vi "save operation binary.vi"(8 "error in":errorcluster, 11 "state cluster":T1) -> (0 "error out":errorcluster, 3 "state out":T1)   [LabVIEW 2013, in "configuration library.lvlib"]
uses:
  configuration library.lvlib
  Controls/StateCluster.ctl
  <vilib>/NI/Tag Bus Data Framework/Configuration Editor/Classes/SystemConfigRepo/SystemConfigRepo.lvclass
  <vilib>/NI/Configuration Framework/Node/NodeRef.ctl
  <vilib>/NI/Configuration Framework/Node/NISE_CEF_Node.lvclass
  <vilib>/NI/Configuration Framework/Node/UserEventRef.ctl
  <vilib>/NI/Configuration Framework/Controls/EventCluster.ctl
  SplashScreen/splash screen.ctl
  SplashScreen/notifier data.ctl
  <vilib>/NI/Configuration Framework/hierarchy repo/NISE_CEF_HierarchyRepo.lvclass
  <vilib>/NI/Configuration Framework/tree serializer/NISE_CEF_TreeSerializer.lvlib
  <vilib>/NI/Configuration Framework/NISE_CEF_TreeControl.lvlib
  SplashScreen/splash screen.lvlib
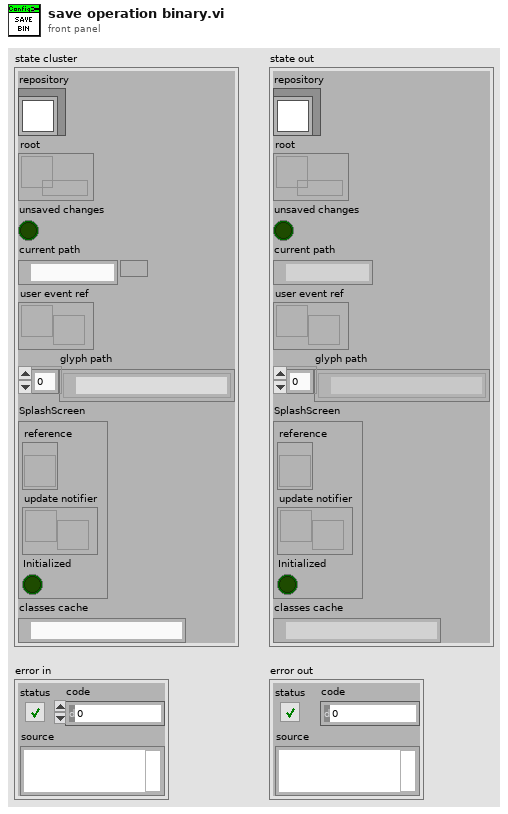
[diagram p1: front panel]
types:
  T1 = typedef "configuration library.lvlib/StateCluster.ctl" = cluster{"repository":refnum<class "SystemConfigRepo.lvclass">, "root":T2, "unsaved changes":bool, "current path":path, "user event ref":T3, "glyph path":path[], "SplashScreen":T4, "classes cache":path}
  T2 = typedef "NISE_CEF_Node.lvclass/NodeRef.ctl" = refnum<data-value>
  T3 = typedef "NISE_CEF_Node.lvclass/UserEventRef.ctl" = refnum<user-event>
  T4 = typedef "configuration library.lvlib/splash screen.lvlib/splash screen.ctl" = cluster{"reference":refnum<vi>, "update notifier":refnum<notifier>, "Initialized":bool}
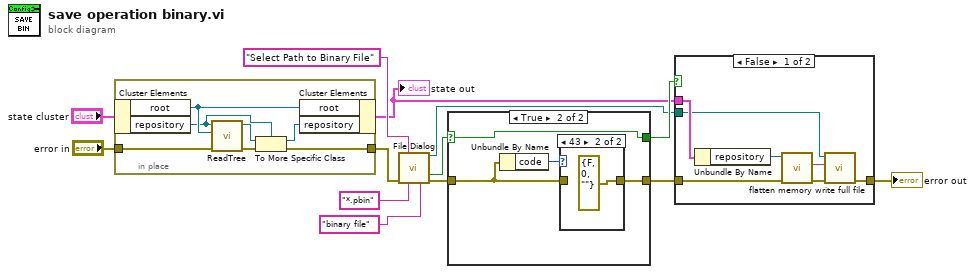
[diagram p0: block diagram]
diagram:
  n1 = in-place {
    in-place-border: "error in" -> [w20]
    in-place-border: [w17] -> w13
    n2 = in-place-cluster #1("state cluster") -> ("root"=w19:T2, "repository"=w15:refnum<class "SystemConfigRepo.lvclass">)
    n3 = call-dynamic "ReadTree.vi"("error in"=w20, "root"=w19, "repository in"=w15) -> ("error out"=w18:errorcluster, "repository out"=w16:refnum<class "NISE_CEF_Repository.lvclass">)  [unwired: 7 in]
    n4 = To More Specific Class(target class=w15, reference=w16, error in=w18) -> (specific class reference=w14:refnum<class "SystemConfigRepo.lvclass">, error out=w17:errorcluster)
    n5 = in-place-cluster #1("root"=w19, "repository"=w14) -> (w1:T1)
  }
  "state out" <- w1
  n6 = call "File Dialog"("prompt"="Select Path to Binary File" ("Prompt"), "error in"=w13, "pattern (all files)"="*.pbin" ("pattern"), "pattern label"="binary file") -> ("selected path"=w8:path, "cancelled"=w3:bool, "error out"=w2:errorcluster)  [unwired: 8 in, 1 out]
  n7 = case shown="True" w3 {
    selector: w3 -> [w21 w23]
    tunnel: w2 -> [w22 w25]
    tunnel: [w22 w24] -> w7
    tunnel: [w21 w23] -> w9
    frame False {
    }
    frame True {
      n8 = Unbundle By Name(w25) -> ("code"=w26:i32)
      n9 = case shown="43" w26 {
        tunnel: w25 -> [w27 _]
        tunnel: [w27 errorcluster {"status"=FALSE, "code"=0, "source"=""} ("error out")] -> w24
        frame Default {
        }
        frame 43 {
        }
      }
    }
  }
  n10 = case shown="False" w9 {
    tunnel: w1 -> [w35 _]
    tunnel: w7 -> [w32 w36]
    tunnel: [w29 w36] -> w12
    tunnel: w8 -> [w31 _]
    frame False {
      n11 = Unbundle By Name(w35) -> ("repository"=w33:refnum<class "SystemConfigRepo.lvclass">)
      n12 = call <vilib>:"flatten memory.vi"("error in"=w32, "NISE_CEF_HierarchyRepo in"=w33) -> ("error out"=w30:errorcluster, "binary repo"=w34:string)  [unwired: 7 in, 1 out]
      n13 = call <vilib>:"write full file.vi"("error in"=w30, "strings"=w34, "file path"=w31) -> ("error out"=w29:errorcluster)  [unwired: 8 in]
    }
    frame True {
    }
  }
  "error out" <- w12
